vi "File Rollover.vi"() -> ()   [LabVIEW 2018]
uses:
  api/Log Levels.ctl
  api/configuration/handlers/file_handler/File Handler.lvclass
  C:/Users/Colin/Documents/software_projects/glog/src/api/extension/formatting_handler_interface/Formatting Handler.lvclass
  api/logger_class/Logger.lvclass
  api/Logging.lvlib
panel:
  in  "delete when done?":bool
  out "error out":errorcluster
  out "2 files? (post-rollover)":bool
  out "1 file? (2nd)":bool
  out "1 file? (1st)":bool
  # "Locals"
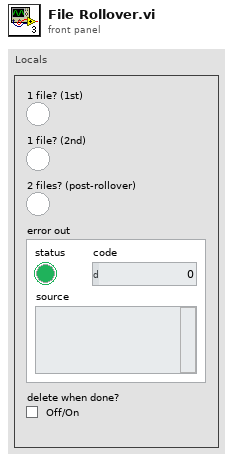
[diagram p1: front panel]
types:
  T1 = typedef "Logging.lvlib/Log Levels.ctl" = enum16{"Trace", "Debug", "Info", "Warning", "Error", "Critical"}
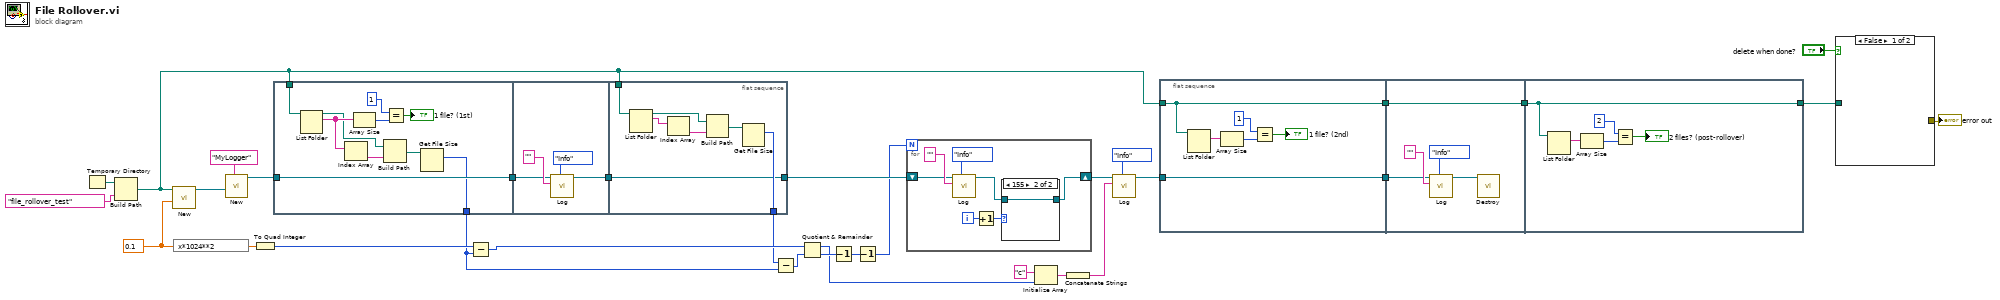
[diagram p0: block diagram]
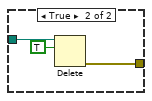
[diagram p3: hidden frame]
diagram:
  w25 = 0.1 ("rollover threshold [MB](50)")
  n1 = Temporary Directory() -> (w30:path)
  n2 = Build Path(base path=w30, name or relative path="file_rollover_test") -> (appended path=w6:path)
  n3 = call "New.vi"("rollover threshold [MB](50)"=w25, "log directory (<app dir>/logs)"=w6) -> ("file handler"=w31:refnum<class "File Handler.lvclass">)  [unwired: 9 in]
  n4 = expression code="x*1024**2"(w25) -> (w13:dbl)
  n5 = call "New.vi"("name (\"Default\")"="MyLogger" ("name"), "log handler (file handler)"=w31) -> ("logger"=w8:refnum<class "Logger.lvclass">)  [unwired: 8 in, 1 out]
  n6 = To Quad Integer(1:w13) -> (0:w5:i64)
  n7 = flat-sequence {
    tunnel: w8 -> [w42]
    tunnel: [w42] -> w7
    tunnel: w6 -> [w35]
    tunnel: [w33] -> w3
    tunnel: [w43] -> w9
    tunnel: w7 -> [w44]
    tunnel: [w50] -> w2
    tunnel: w6 -> [w49]
    tunnel: [w48] -> w16
    tunnel: w9 -> [w48]
    frame #0 {
      n8 = List Folder(path=w35) -> (path out=w37:path, filenames=w39:string[])  [unwired: 3 in, 2 out]
      n9 = Index Array(array=w39) -> (element=w38:string)  [unwired: 1 in]
      n10 = Array Size(array=w39) -> (size(s)=w40:i32)
      n11 = Build Path(base path=w37, name or relative path=w38) -> (appended path=w36:path)
      n12 = Equal?(x=1, y=w40) -> (x = y?=→"1 file? (1st)":bool)
      n13 = Get File Size(file=w36) -> (size (in bytes)=w33:i64)  [unwired: 1 in, 2 out]
    }
    frame #1 {
      n14 = call "Log.vi"("log level"=Log_Levels."Info" ("level"), "message"="", "logger in"=w44) -> ("logger out"=w43:refnum<class "Logger.lvclass">)  [unwired: 8 in]
    }
    frame #2 {
      n15 = List Folder(path=w49) -> (path out=w51:path, filenames=w53:string[])  [unwired: 3 in, 2 out]
      n16 = Index Array(array=w53) -> (element=w52:string)  [unwired: 1 in]
      n17 = Build Path(base path=w51, name or relative path=w52) -> (appended path=w47:path)
      n18 = Get File Size(file=w47) -> (size (in bytes)=w50:i64)  [unwired: 1 in, 2 out]
    }
  }
  n19 = Subtract(x=w5, y=w3) -> (x-y=w4:i64)
  n20 = Subtract(x=w2, y=w3) -> (x-y=w1:i64)
  n21 = Quotient & Remainder(x=w4, y=w1) -> (x-y*floor(x/y)=w18:i64, floor(x/y)=w24:i64)
  n22 = Decrement(x=w24) -> (x-1=w23:i64)
  n23 = Decrement(x=w23) -> (x-1=w15:i64)
  n24 = for {
    N: w15 -> [_]
    shift-right: [w55] -> w22
    shift-left: w16 -> [w57]
    i -> [w58]
    n25 = call "Log.vi"("log level"=Log_Levels."Info" ("level"), "message"="", "logger in"=w57) -> ("logger out"=w56:refnum<class "Logger.lvclass">)  [unwired: 8 in]
    n26 = Increment(x=w58) -> (x+1=w54:i32)
    n27 = case shown="155" w54 {
      tunnel: w56 -> [w61 w62]
      tunnel: [w61 w62] -> w55
      frame Default {
      }
      frame 155 {
      }
    }
  }
  n28 = Initialize Array("c" ("message"), w18) -> (w20:string[])
  n29 = Concatenate Strings(w20) -> (w17:string)
  n30 = call "Log.vi"("log level"=Log_Levels."Info" ("level"), "message"=w17, "logger in"=w22) -> ("logger out"=w11:refnum<class "Logger.lvclass">)  [unwired: 8 in]
  n31 = flat-sequence {
    tunnel: w6 -> [w64]
    tunnel: w11 -> [w65]
    tunnel: [w65] -> w28
    tunnel: [w64] -> w27
    tunnel: w28 -> [w70]
    tunnel: w27 -> [w73]
    tunnel: [w73] -> w26
    tunnel: w26 -> [w75]
    tunnel: [w75] -> w14
    frame #0 {
      n32 = List Folder(path=w64) -> (filenames=w68:string[])  [unwired: 3 in, 3 out]
      n33 = Array Size(array=w68) -> (size(s)=w67:i32)
      n34 = Equal?(x=1, y=w67) -> (x = y?=→"1 file? (2nd)":bool)
    }
    frame #1 {
      n35 = call "Log.vi"("log level"=Log_Levels."Info" ("level"), "message"="", "logger in"=w70) -> ("logger out"=w69:refnum<class "Logger.lvclass">)  [unwired: 8 in]
      n36 = call "Destroy.vi"("logger in"=w69) -> ()  [unwired: 9 in, 2 out]
    }
    frame #2 {
      n37 = List Folder(path=w75) -> (filenames=w78:string[])  [unwired: 3 in, 3 out]
      n38 = Array Size(array=w78) -> (size(s)=w77:i32)
      n39 = Equal?(x=2, y=w77) -> (x = y?=→"2 files? (post-rollover)":bool)
    }
  }
  n40 = case shown="False" "delete when done?" {
    tunnel: w14 -> [_ w80]
    tunnel: [_ w79] -> w12
    frame False {
    }
    frame True {
      n41 = Delete(path (use dialog)=w80, entire hierarchy (F)=TRUE) -> (error out=w79:errorcluster)  [unwired: 3 in, 2 out]
    }
  }
  "error out" <- w12
